vi "ExADCAsync.vi"() -> ()   [LabVIEW 2010]
uses:
  Open-Close/CamHandle.vi
panel:
  in  "Intensifier":bool
  out "Pixel Time":i32
  out "Bit Depth":i32
  out "ReadOut port":i32
  out "ADC Offset":i32
  out "ADC Gain":i32
  out "ADC Speed":i32
  in  "Readout Port":i32=-1 min=-1 step=1
  in  "ADC Offset":i32=-1 min=-1 step=1
  in  "ADC Gain":i32=-1 min=-1 step=1
  in  "ADC speed":i32=-2 min=-3 step=1
  in  "Trigger Edge":u32(ring)=1 items=["N/A", "Positive (leading) edge", "Negative (falling) edge"]
  in  "Timing Mode":u32(ring)=1 items=["N/A", "Free Run/Timed", "Trigger First (PM only)", "Ext Sync/Strobed ", "Variable Exp (PM only)", "Flash Mode (PM only)"]
  in  "Temperature":dbl format="%.2f"
  in  "Exposure":dbl min=0.0 step=0.001 format="%.3f"
  in  "stop":bool
  in  "Store":bool
  out "error out":errorcluster
  in  "error in (no error)":errorcluster
  # "ExADCAsync:\nThis program shows how to use the  CameraADCset.vi and the CameraADCget.vi. This example allows all the ADC settings to be set or ignored."
  # "The following are read \nfrom camera after setting\nvalues to left.\n-1 value means it isn't \nsupported by camera."
  # "For Slowest ADC speed set this to -3\nFor Fastest ADC speed set this to -2\nTo use current ADC speed don't  hook up or use -1\notherwise put speed in as kHz"
  # "To use current gain don't hook up or set to -1"
  # "To use current gain don't hook up or set to -1"
  # "To use current gain don't hook up or set to -1"
  # "NOTICE\n\nTHIS VI USES A GLOBAL CAMERA HANDLE\n\nTHE VI EXOPENGLOBALCAM.VI MUST BE\nRUN AT THE START OF THE WORK SESSION.\nTHE CAMERA WILL REMAIN OPENED.\n\nTHE VI EXCLOSEGLOBALCAM.VI MUST\nBE RUN BEFORE LEAVING LABVIEW."
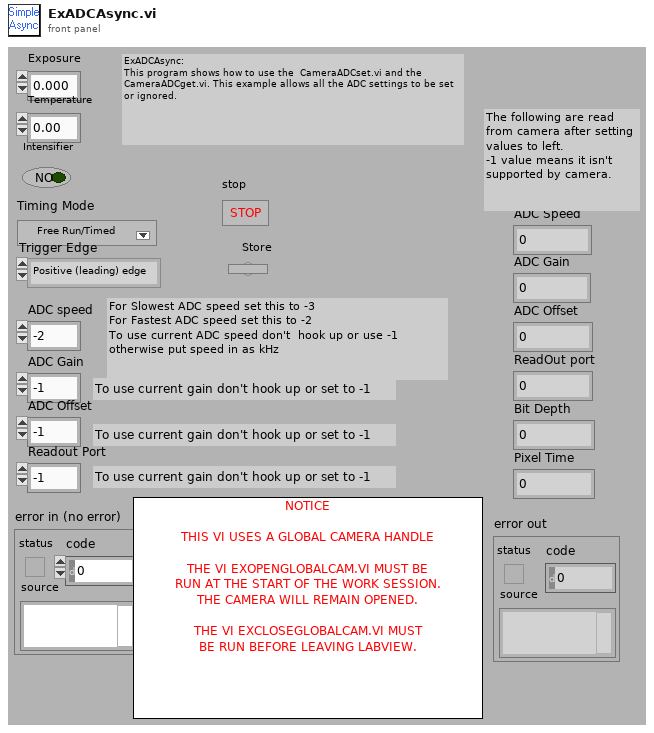
[diagram p1: front panel]
types:
  T1 = cluster{"Acquire mode \n3 is Async":i32, "Exposure":dbl, "Number of Images":i32, "Software Accums":i32}
  T2 = cluster{"Camera Handle":u32, "Pulser Handle":u32, "File Handle":u32, "Display Handle":u32, "Image Handle":u32}
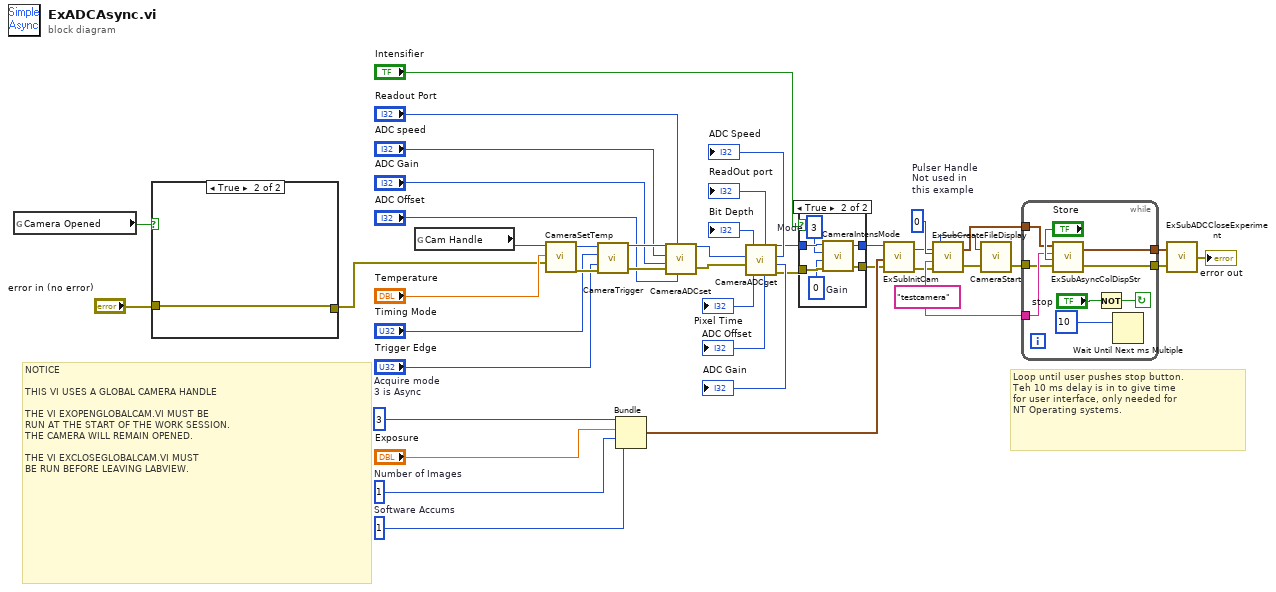
[diagram p0: block diagram]
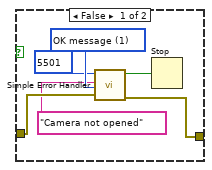
[diagram p2: hidden frame]
diagram:
  w36 = 0  # Pulser Handle Not used in  this example
  w41 = 1  # Number of Images
  w42 = 3  # Acquire mode  3 is Async
  w40 = 1  # Software Accums
  w43 = "testcamera"
  # "NOTICE\n\nTHIS VI USES A GLOBAL CAMERA HANDLE\n\nTHE VI EXOPENGLOBALCAM.VI MUST BE\nRUN AT THE START OF THE WORK SESSION.\nTHE CAMERA WILL REMAIN OPENED.\n\nTHE VI EXCLOSEGLOBALCAM.VI MUST\nBE RUN BEFORE LEAVING LABVIEW."
  # "Loop until user pushes stop button.\nTeh 10 ms delay is in to give time \nfor user interface, only needed for \nNT Operating systems."
  n1 = global read "CamHandle.vi" "Camera Opened"() -> (w4:bool)
  n2 = case shown="True" w4 {
    tunnel: "error in (no error)" -> [w48 w50]
    tunnel: [w47 w50] -> w2
    frame False {
      w49 = u16 1 items=["no dialog", "OK message", "continue or stop message"] ("type of dialog (OK msg:1)")
      n3 = call <vilib>:"Simple Error Handler.vi"("error code (no error:0)"=5501, "error source (\" \")"="Camera not opened", "type of dialog (OK msg:1)"=w49, "error in (no error)"=w48) -> ("error?"=w45:bool, "error out"=w47:errorcluster)  [unwired: 1 in, 3 out]
      n4 = Stop(stop? (T)=w45) -> ()
    }
    frame True {
    }
  }
  n5 = global read "CamHandle.vi" "Cam Handle"() -> (w1:u32)
  n6 = call <userlib>:"CameraSetTemp.vi"("error in (no error)"=w2, "Temperature"="Temperature", "Camera Handle"=w1) -> ("error out"=w26:errorcluster, "Camera Handle"=w27:u32)
  n7 = call <userlib>:"CameraTrigger.vi"("error in"=w26, "Trigger Edge"="Trigger Edge", "Timing Mode"="Timing Mode", "Camera Handle"=w27) -> ("error out"=w14:errorcluster, "Camera Handle"=w15:u32)
  n8 = Bundle("Acquire mode \n3 is Async"=w42, "Exposure"="Exposure", "Number of Images"=w41, "Software Accums"=w40) -> (w38:T1)  [unwired: 1 in]
  n9 = call <userlib>:"CameraADCset.vi"("ADC offset"="ADC Offset", "Read Out port"="Readout Port", "error in (no error)"=w14, "ADC Gain"="ADC Gain", "ADC Speed"="ADC speed", "Camera Handle"=w15) -> ("error out"=w17:errorcluster, "Camera Handle"=w18:u32)
  n10 = call <userlib>:"CameraADCget.vi"("Camera handle"=w18, "error in (no error)"=w17) -> ("Bit Depth"=→"Bit Depth":i32, "Pixel Time"=→"Pixel Time":i32, "Readout Port"=→"ReadOut port":i32, "ADC Offset"=→"ADC Offset":i32, "Camera handle"=w6:u32, "ADC Speed"=→"ADC Speed":i32, "ADC Gain"=→"ADC Gain":i32, "error out"=w7:errorcluster)
  n11 = case shown="True" "Intensifier" {
    tunnel: w6 -> [w52 w58]
    tunnel: [w52 w57] -> w8
    tunnel: w7 -> [w51 w56]
    tunnel: [w51 w55] -> w9
    frame False {
    }
    frame True {
      w53 = u32 0  # Gain
      w54 = u32 3  # Mode
      n12 = call <userlib>:"CameraIntensMode.vi"("error in"=w56, "Intensifier Gain"=w53, "Mode"=w54, "Camera Handle"=w58) -> ("error out"=w55:errorcluster, "Camera Handle"=w57:u32)
    }
  }
  n13 = call "ExSubInitCam.vi"("error in (no error)"=w9, "Camera Information"=w38, "Camera Handle"=w8) -> ("error out"=w37:errorcluster, "Camera Handle"=w32:u32)
  n14 = call "ExSubCreateFileDisplay.vi"("error in (no error)"=w37, "File and Display Name"=w43, "Pulser Handle"=w36, "Camera Handle"=w32) -> ("error out"=w35:errorcluster, "Handles Out"=w34:T2)
  n15 = call <userlib>:"CameraStart.vi"("error in"=w35, "Camera Handle"=w32) -> ("error out"=w33:errorcluster)  [unwired: 1 out]
  n16 = while {
    tunnel: w34 -> [w65]
    tunnel: w33 -> [w63]
    tunnel: w43 -> [w64]
    tunnel: [w61] -> w30
    tunnel: [w62] -> w31
    stop <- w60 continue-if-true
    n17 = call "ExSubAsyncColDispStr.vi"("error in (no error)"=w63, "Store Data"="Store", "Display Title"=w64, "Handle Cluster"=w65) -> ("error out"=w61:errorcluster, "Handle Cluster Out"=w62:T2)
    n18 = Not(x="stop") -> (.not. x?=w60:bool)
    n19 = Wait Until Next ms Multiple(millisecond multiple=10) -> ()  [unwired: 1 out]
  }
  n20 = call "ExSubADCCloseExperiment.vi"("error in (no error)"=w30, "Handles In"=w31) -> ("error out"=→"error out":errorcluster)
